vi "Program_Active.vi"(0 "Hit Server Now":bool) -> ()   [LabVIEW 2017]
uses:
  ADAM Controls/Traverse_Level_State.ctl
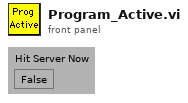
[diagram p1: front panel]
types:
  T1 = typedef "Traverse_Level_State.ctl" = enum16{"Running", "Complete"}
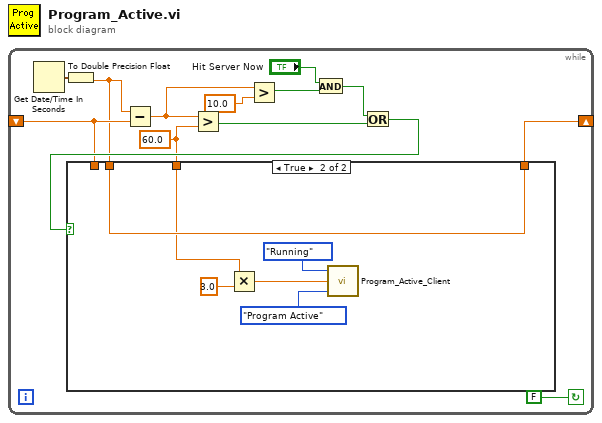
[diagram p0: block diagram]
diagram:
  n1 = while {
    shift-left: _ -> [w10]
    shift-right: [w11] -> _
    stop <- FALSE continue-if-true
    w1 = 60.0 ("y")
    n2 = Get Date/Time In Seconds() -> (seconds since 1Jan1904=w2:timestamp)
    n3 = To Double Precision Float(number=w2) -> (double precision float=w9:dbl)
    n4 = Subtract(x=w9, y=w10) -> (x-y=w8:dbl)
    n5 = Greater?(x=w8, y=w1) -> (0:w13:bool)
    n6 = Greater?(x=w8, y=10.0) -> (0:w5:bool)
    n7 = And(x="Hit Server Now", y=w5) -> (x .and. y?=w4:bool)
    n8 = Or(x=w4, y=w13) -> (x .or. y?=w12:bool)
    n9 = case shown="True" w12 {
      tunnel: [w14 w19] -> w11
      tunnel: w9 -> [_ w19]
      tunnel: w10 -> [w14 _]
      tunnel: w1 -> [_ w17]
      frame False {
      }
      frame True {
        n10 = Multiply(x=w17, y=3.0) -> (x*y=w15:dbl)
        n11 = call "Program_Active_Client.vi"("Mode"=enum16{"Program Active", "Traverse Level State"}."Program Active", "Time till next contact (Sec)"=w15, "Traverse level State"=Traverse_Level_State."Running") -> ()  [unwired: 3 out]
      }
    }
  }
